vi "Get Registration Number.vi"(7 "등록번호 List 참조":refnum<vi>, 8 "에러 입력(에러 없음)":errorcluster, 11 "기기번호":string) -> (0 "에러 출력":errorcluster)   [LabVIEW 2020]
uses:
  Controls/Cmd_Read Query.ctl
  Controls/Clst_Query Info.ctl
  Public/Polymorph/Cell Space_ListBox.vi
  <vilib>/addons/database/NI_Database_API.lvlib
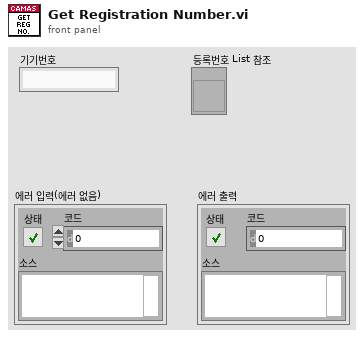
[diagram p1: front panel]
types:
  T1 = typedef "Clst_Query Info.ctl" = cluster{"사번":string, "등록번호":string, "업체명":string, "세부분류코드":string, "형식":string, "기기번호":string, "FUNC":string, "FUNC_EXT":string, "옵션":string, "추가문자열":string, "일자":string, "배열 1":string[], "배열 2":string[], "항목명":string, "문자열":string, "이름":string}
  T2 = typedef "Cmd_Read Query.ctl" = enum16{"교정자 이름 얻기", "인증교정자 얻기", "기술책임자 얻기", "기책부책 얻기", "등록번호 얻기", "등록정보 얻기", "업체정보 얻기", "교정일자(CAMAS) 얻기", "교정일자(CALSTD) 얻기", "교정환경 얻기", "교정절차서 목록 얻기", "교정절차서명 얻기", "교정절차 목록얻기", "교정절차 얻기", "PROC 교정절차 얻기", "PROC SPEC 얻기", "교정절차(Func별) 얻기", "교정절차(Func_ext별) 얻기", "기관코드 얻기", "교정기능(세부분류) 얻기", "교정기능(모델) 얻기", "교정기능 목록 얻기", "교정기능 명칭 얻기", "교정기능 항목명칭 얻기", "DB (사용기준기) 얻기", "DB (기준기이름) 얻기", "DB (기준기이름목록) 얻기", "DB (기준기목록) 얻기", "DB (기준기값) 얻기", "DB (CMC) 얻기", "DB (FUNC) 얻기", "DB (CALNAME) 얻기", "DB (STDNAME) 얻기", "DB (SPEC) 얻기", "모델(항목전체) 얻기", "모델(최대범위) 얻기", "모델(최소범위) 얻기", "모델(최대최소) 얻기", "모델(범위조건) 얻기", "모델(등록요청) 얻기", "모델(형식별) 얻기", "모델(조건별) 얻기", "모델(모델검색) 얻기", "세부분류 목록 얻기", "기준기등록리스트 얻기", "STD Cal Date Check", "DB등록일자 얻기", "적용항목 얻기", "기타정보 얻기", "기준기요청 얻기", "서버버전 얻기"}
  T3 = typedef "NI_Database_API.lvlib/Conn ObjectReference.ctl" = refnum<k1>
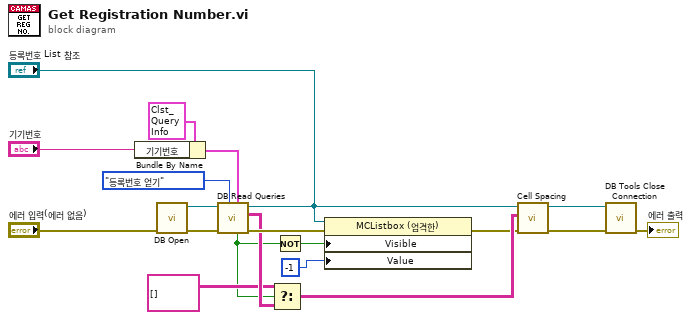
[diagram p0: block diagram]
diagram:
  n1 = Bundle By Name(cluster=T1 {"사번"="", "등록번호"="", "업체명"="", "세부분류코드"="", "형식"="", "기기번호"="", "FUNC"="", "FUNC_EXT"="", "옵션"="", "추가문자열"="", "일자"="", "배열 1"=[], "배열 2"=[], "항목명"="", "문자열"="", "이름"=""} ("Query info"), "기기번호"="기기번호") -> (w18:T1)
  n2 = call "DB Open.vi"("에러 입력"="에러 입력(에러 없음)") -> ("에러 출력"=w12:errorcluster, "참조 번호 출력"=w13:T3)  [unwired: 9 in]
  n3 = call "DB Read Queries.vi"("Query info"=w18, "Query Command"=Cmd_Read_Query."등록번호 얻기", "에러 입력(에러 없음)"=w12, "참조 번호 입력"=w13) -> ("에러 출력"=w16:errorcluster, "Data"=w8:string[][], "참조 번호 출력"=w14:T3, "None?"=w5:bool)  [unwired: 3 in, 1 out]
  n4 = Select(t=string[][] [], s=w5, f=w8) -> (s? t:f=w3:string[][])
  n5 = Not(x=w5) -> (.not. x?=w6:bool)
  n6 = property on="프로퍼티 노드" class="MCListbox (엄격한)"(reference="등록번호 List 참조", error in=w16, "Visible"=w6, "Value"=-1 ("등록번호 List")) -> (error out=w2:errorcluster)  [unwired: 1 out]
  n7 = call-poly "Cell Spacing.vi"("error in"=w2, "Data in"=w3, "여러열리스트박스 참조 in"="등록번호 List 참조") -> ("error out"=w1:errorcluster)  [unwired: 7 in, 1 out]
  n8 = call <vilib>:"DB Tools Close Connection.vi"("error in (no error)"=w1, "connection reference"=w14) -> ("error out"=→"에러 출력":errorcluster)  [unwired: 5 in]
